vi "macro_LTV_DiffDriveCtrl_Execute.vi"() -> ()   [LabVIEW 2019, in "Trajectory_Library.lvlib"]
uses:
  Trajectory_Library.lvlib
  TypeDef/POSE2D.ctl
  TypeDef/TRANSLATION2D.ctl
  TypeDef/ROTATION2D.ctl
  Enum/DCMOTOR_TYPES_ENUM.ctl
  Enum/DIFF_DRIVE_ToughBoxMini_GearChoice_ENUM.ctl
  LinearSystemId_CreateDriveTrainVelocitySystem.vi
  DCMotor_PickMotor.vi
  LinearSystem_New.vi
  MatBuilder_Create.vi
  MatBuilder_Fill.vi
  MatrixHelper_Zero.vi
  DCMotor_GetCIM.vi
  DCMotor_GetAndymark9015.vi
  DCMotor_GetAndymarkRs775_125.vi
  DCMotor_GetBag.vi
  DCMotor_GetBanebotsRs550.vi
  DCMotor_GetBanebotsRs775.vi
  DCMotor_GetFalcon500.vi
  DCMotor_GetMiniCIM.vi
  DCMotor_GetNEO.vi
  DCMotor_GetNEO550.vi
  DCMotor_GetRomiBuiltIn.vi
  DCMotor_GetVex775Pro.vi
  VI/DCMotor_GetAndymarkAM2235A.vi
  VI/DCMotor_GetAndymarkAM3493.vi
  MatrixHelper_CoerceSize.vi
  DCMotor_New.vi
  VI/Units_RotationsPerMinuteToRadiansPerSecond.vi
panel:
  in  "Right Velocity":dbl
  in  "Left Velocity":dbl
  in  "Ref Right Velocity":dbl
  in  "Ref Left Velocity":dbl
  out "Right Motor Dmd":dbl
  out "Left Motor Dmd":dbl
  in  "CurrentPose":T1={"TRANSLATION"={"X"=0.0, "Y"=0.0}, "ROTATION"={"VALUE"=0.0, "COS"=1.0, "SIN"=0.0}} {"ROTATION"."SIN" format="%13.4f"; "ROTATION"."COS" format="%13.4f"; "ROTATION"."VALUE" format="%13.4f"; "TRANSLATION"."Y" format="%14.3f"; "TRANSLATION"."X" format="%14.3f"}
  in  "RefPose":T1={"TRANSLATION"={"X"=0.0, "Y"=0.0}, "ROTATION"={"VALUE"=0.0, "COS"=1.0, "SIN"=0.0}} {"ROTATION"."SIN" format="%13.4f"; "ROTATION"."COS" format="%13.4f"; "ROTATION"."VALUE" format="%13.4f"; "TRANSLATION"."Y" format="%14.3f"; "TRANSLATION"."X" format="%14.3f"}
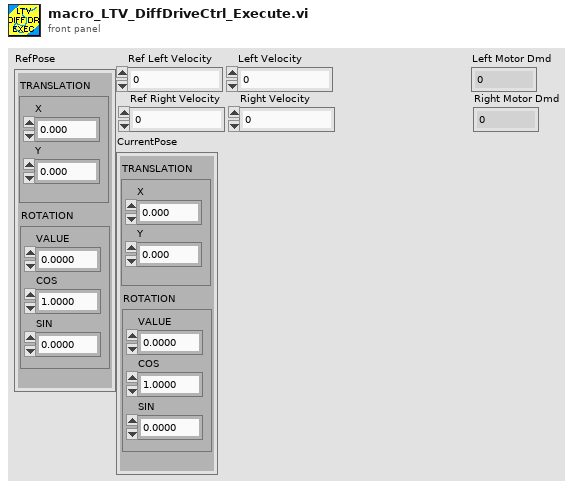
[diagram p1: front panel]
types:
  T1 = typedef "Trajectory_Library.lvlib/POSE2D.ctl" = cluster{"TRANSLATION":T2, "ROTATION":T3}
  T2 = typedef "Trajectory_Library.lvlib/TRANSLATION2D.ctl" = cluster{"X":dbl, "Y":dbl}
  T3 = typedef "Trajectory_Library.lvlib/ROTATION2D.ctl" = cluster{"VALUE":dbl, "COS":dbl, "SIN":dbl}
  T4 = typedef "Trajectory_Library.lvlib/DIFF_DRIVE_ToughBoxMini_GearChoice_ENUM.ctl" = enum16{"Ratio_12_75", "Ratio_10_71", "Ratio_8_45", "Ratio_7_31", "Ratio_5_95"}
  T5 = typedef "Trajectory_Library.lvlib/DCMOTOR_TYPES_ENUM.ctl" = enum16{"CIM", "AndyMark 9015", "Andy Mark RS 775 125", "Bag", "BaneBots RS 550", "BaneBots RS 775", "Falcon 500", "Mini CIM", "NEO", "NEO 550", "Romi BuiltIn", "Vex 775 Pro", "Snow Blower AM 2235A", "Bosch Seat AM 3493"}
  T6 = typedef "Trajectory_Library.lvlib/LINEAR_SYSTEM.ctl" = cluster{"m_A":T7, "m_B":T7, "m_C":T7, "m_D":T7, "States":i32, "Inputs":i32, "Outputs":i32}
  T7 = typedef "NI_Matrix.lvlib/RealMatrix.ctl" = dbl[][]
  T8 = typedef "Trajectory_Library.lvlib/LTV_DIFF_DRIVE_CTRL_TOLERANCE.CTL" = cluster{"Max Heading Tolerance Rad":dbl, "Max X Tolerance M":dbl, "Max Y Tolerance M":dbl, "Max Left Vel Tol M/S":dbl, "Max Right Vel Tol M/S":dbl}
  T9 = typedef "LTV_DIFF_DRIVE_CTRL_CONTROL_PARAMS.CTL" = cluster{"Max left vel ctrl effort V":dbl, "Desired Heading Ctrl Tol Rad":dbl, "Desired Y Pos Meas Tol M":dbl, "Desired X Pos Ctrl Tol M":dbl, "Desired Left Vel Ctrl Tol M/S":dbl, "Desired Right Vel Ctrl Tol M/S":dbl, "Max right vel ctrl effort V":dbl}
  T10 = typedef "Trajectory_Library.lvlib/LTV_DIFF_DRIVE_CTRL_MODEL_PARAMS.CTL" = cluster{"Track Width":dbl, "Diff_Drive_Linear_System":T6, "LTV_DiffDriveCtrl_Control":T9, "LTV_DiffDriveCtrl_Tolerance":T8, "dT Sec":dbl}
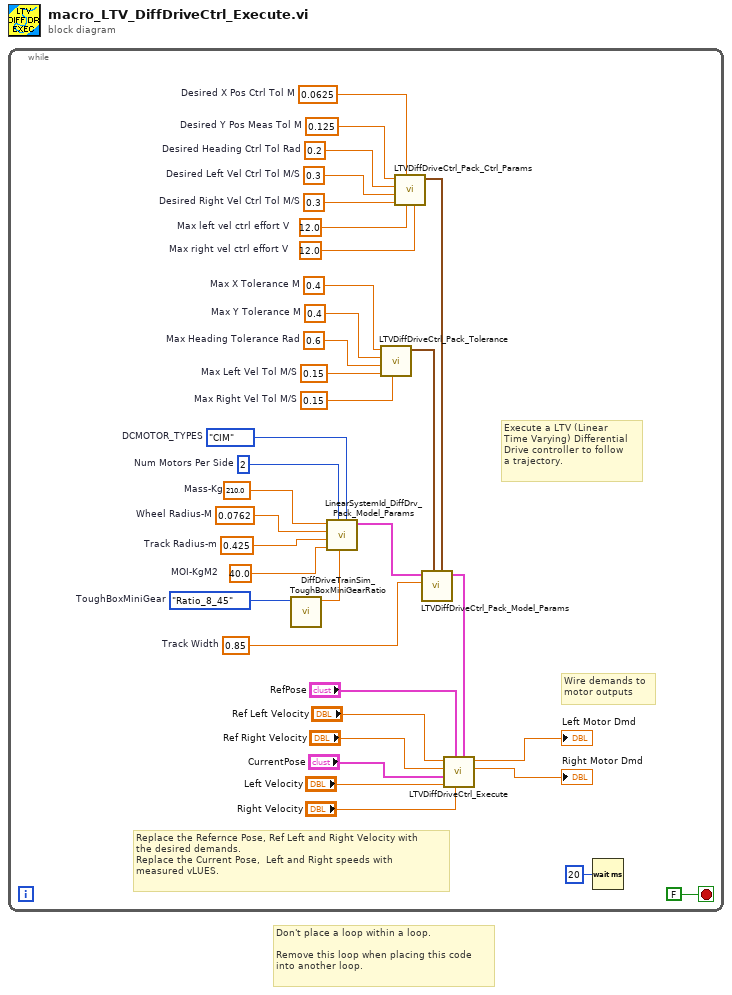
[diagram p0: block diagram]
diagram:
  # "Don't place a loop within a loop.\n \nRemove this loop when placing this code\ninto another loop."
  n1 = while {
    stop <- FALSE stop-if-true
    w2 = DIFF_DRIVE_ToughBoxMini_GearChoice_ENUM."Ratio_8_45"  # ToughBoxMiniGear
    w3 = 210.0  # Mass-Kg
    w4 = 0.0762  # Wheel Radius-M
    w5 = 0.425  # Track Radius-m
    w6 = 40.0  # MOI-KgM2
    w7 = 2  # Num Motors Per Side
    w8 = DCMOTOR_TYPES_ENUM."CIM"  # DCMOTOR_TYPES
    w10 = 0.4  # Max X Tolerance M
    w11 = 0.4  # Max Y Tolerance M
    w12 = 0.6  # Max Heading Tolerance Rad
    w13 = 0.15  # Max Left Vel Tol M/S
    w14 = 0.15  # Max Right Vel Tol M/S
    w15 = 0.125  # Desired Y Pos Meas Tol M
    w16 = 0.2  # Desired Heading Ctrl Tol Rad
    w17 = 0.3  # Desired Left Vel Ctrl Tol M/S
    w18 = 0.3  # Desired Right Vel Ctrl Tol M/S
    w19 = 0.0625  # Desired X Pos Ctrl Tol M
    w20 = 12.0  # Max left vel ctrl effort V
    w21 = 12.0  # Max right vel ctrl effort V
    w30 = 0.85  # Track Width
    # "Wire demands to\nmotor outputs"
    # "Replace the Refernce Pose, Ref Left and Right Velocity with \nthe desired demands.\nReplace the Current Pose,  Left and Right speeds with\nmeasured vLUES."
    # "Execute a LTV (Linear \nTime Varying) Differential \nDrive controller to follow\na trajectory."
    n2 = call "DiffDriveTrainSim_ToughBoxMiniGearRatio.vi"("ToughBoxMiniGear"=w2) -> ("GearRatio"=w1:dbl)  [unwired: 10 in]
    n3 = call "LinearSystemId_DiffDrv_Pack_Model_Params.vi"("DCMOTOR_TYPES"=w8, "Gear Ratio"=w1, "Num Motors Per Side"=w7, "MOI-KgM2"=w6, "Track Radius-m"=w5, "Wheel Radius-M"=w4, "Mass-Kg"=w3) -> ("DiffDrv_LinearSystem"=w9:T6)  [unwired: 4 in]
    n4 = call "LTVDiffDriveCtrl_Pack_Tolerance.vi"("Max Right Vel Tol M/S"=w14, "Max Left Vel Tol M/S"=w13, "Max Heading Tolerance Rad"=w12, "Max Y Tolerance M"=w11, "Max X Tolerance M"=w10) -> ("LTV_DiffDriveCtrl_Tolerance"=w31:T8)  [unwired: 6 in]
    n5 = call "LTVDiffDriveCtrl_Pack_Ctrl_Params.vi"("Max right vel ctrl effort V"=w21, "Max left vel ctrl effort V"=w20, "Desired X Pos Ctrl Tol M"=w19, "Desired Right Vel Ctrl Tol M/S"=w18, "Desired Left Vel Ctrl Tol M/S"=w17, "Desired Heading Ctrl Tol Rad"=w16, "Desired Y Pos Meas Tol M"=w15) -> ("LTV_DiffDriveCtrl_Control"=w32:T9)  [unwired: 4 in]
    n6 = call "LTVDiffDriveCtrl_Pack_Model_Params.vi"("LTV_DiffDriveCtrl_Control"=w32, "LTV_DiffDriveCtrl_Tolerance"=w31, "Track Width"=w30, "Diff_Drive_Linear_System"=w9) -> ("LTV_DiffDriveCtrl_Model"=w33:T10)  [unwired: 7 in]
    n7 = call "LTVDiffDriveCtrl_Execute.vi"("LTV_DiffDriveCtrl_Model"=w33, "Right Velocity"="Right Velocity", "RefPose"="RefPose", "Left Velocity"="Left Velocity", "CurrentPose"="CurrentPose", "Ref Right Velocity"="Ref Right Velocity", "Ref Left Velocity"="Ref Left Velocity") -> ("Right Motor Dmd"=→"Right Motor Dmd":dbl, "Left Motor Dmd"=→"Left Motor Dmd":dbl)  [unwired: 3 out]
    n8 = Wait (ms)(milliseconds to wait=u32 20) -> ()  [unwired: 1 out]
  }
